vi "new DSF Configuration.vi"(8 "error in (no error)":errorcluster) -> (0 "error out":errorcluster, 3 "configuration cluster":T1)   [LabVIEW 2017, in "DSF Configuration API v1.0.0.lvlib"]
uses:
  DSF Configuration API v1.0.0.lvlib
  Controls/dsf configuration data/1.0.0/dsf configuration.ctl
  Controls/dsf configuration data/1.0.0/version.ctl
  Controls/dsf configuration data/1.0.0/dsf plugin.ctl
  Controls/dsf configuration data/1.0.0/dsf timing.ctl
  Controls/dsf configuration data/1.0.0/dsf group.ctl
  Controls/dsf configuration data/1.0.0/dsf transfer.ctl
  Controls/dsf configuration data/1.0.0/dsf channel.ctl
  Controls/dsf configuration data/1.0.0/dsf settings.ctl
  Controls/dsf configuration data/1.0.0/dsf configuration data v1.0.0.lvlib
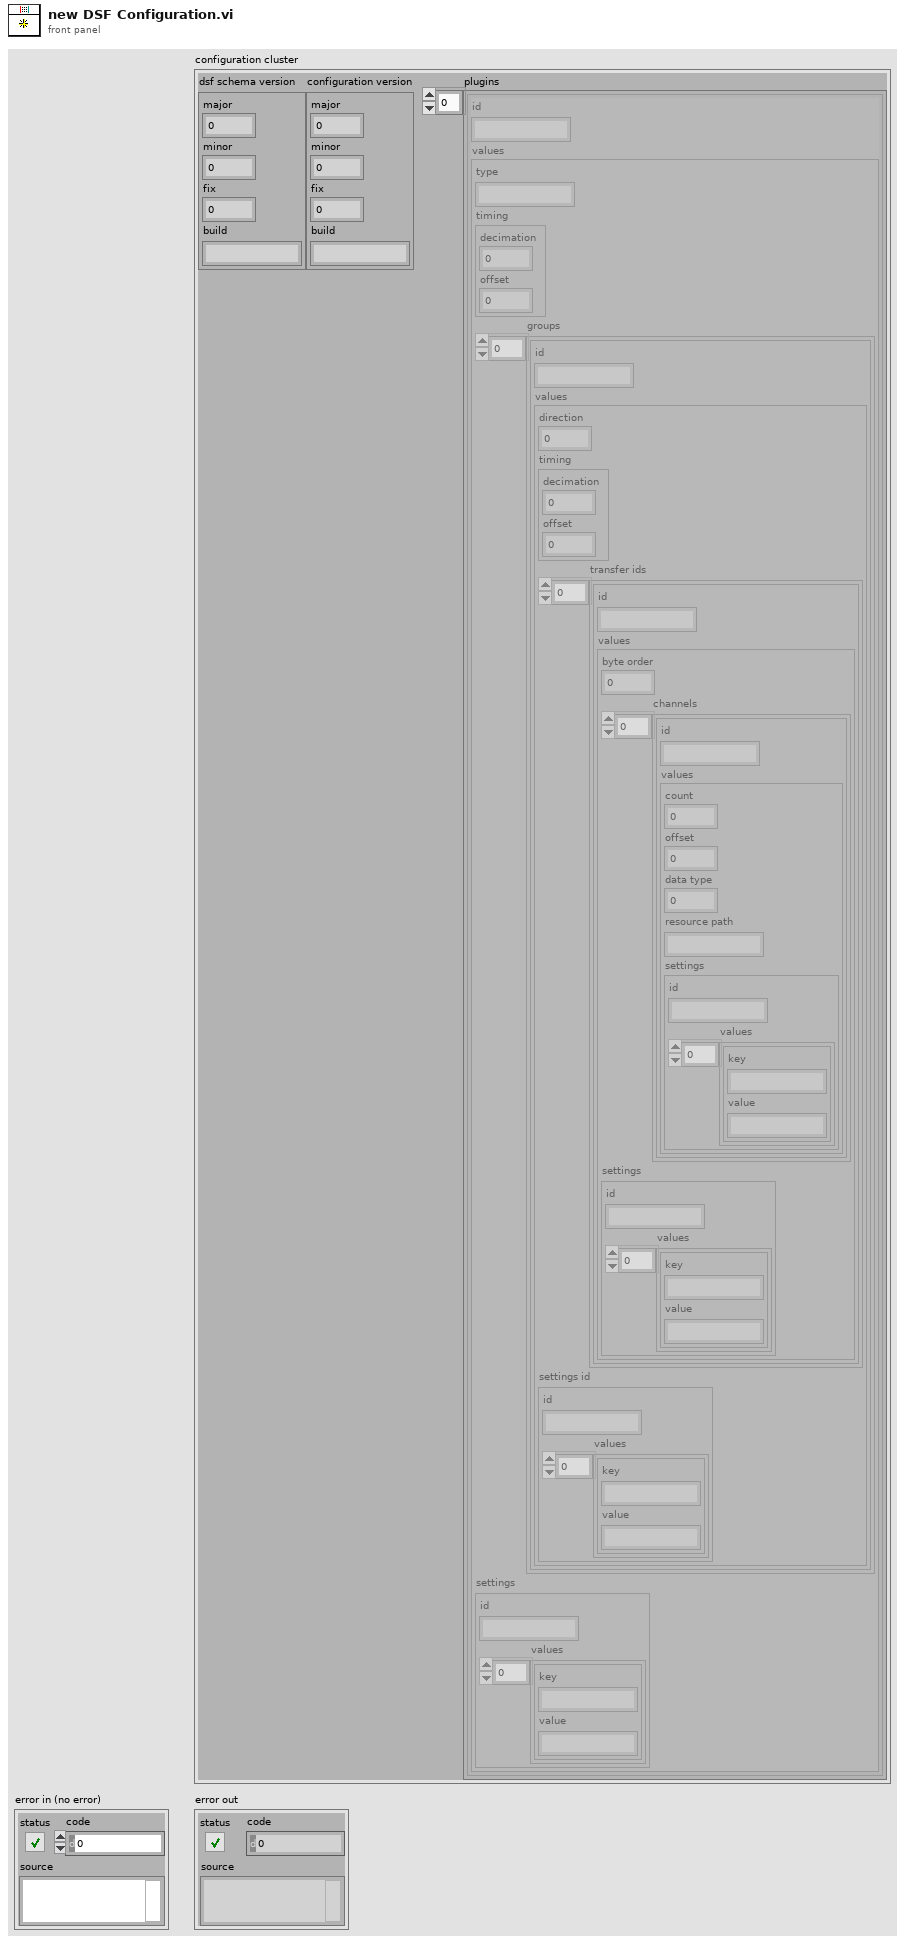
[diagram p1: front panel]
types:
  T1 = typedef "dsf configuration data v1.0.0.lvlib/dsf configuration.ctl" = cluster{"dsf schema version":T2, "configuration version":T2, "plugins":T3[]}
  T2 = typedef "dsf configuration data v1.0.0.lvlib/version.ctl" = cluster{"major":u32, "minor":u32, "fix":u32, "build":string}
  T3 = typedef "dsf configuration data v1.0.0.lvlib/dsf plugin.ctl" = cluster{"id":string, "values":cluster{"type":string, "timing":T4, "groups":T5[], "settings":T8}}
  T4 = typedef "dsf configuration data v1.0.0.lvlib/dsf timing.ctl" = cluster{"decimation":i32, "offset":i32}
  T5 = typedef "dsf configuration data v1.0.0.lvlib/dsf group.ctl" = cluster{"id":string, "values":cluster{"direction":i32, "timing":T4, "transfer ids":T6[], "settings id":T8}}
  T6 = typedef "dsf configuration data v1.0.0.lvlib/dsf transfer.ctl" = cluster{"id":string, "values":cluster{"byte order":i32, "channels":T7[], "settings":T8}}
  T7 = typedef "dsf configuration data v1.0.0.lvlib/dsf channel.ctl" = cluster{"id":string, "values":cluster{"count":i32, "offset":i32, "data type":i32, "resource path":string, "settings":T8}}
  T8 = typedef "dsf configuration data v1.0.0.lvlib/dsf settings.ctl" = cluster{"id":string, "values":cluster{"key":string, "value":string}[]}
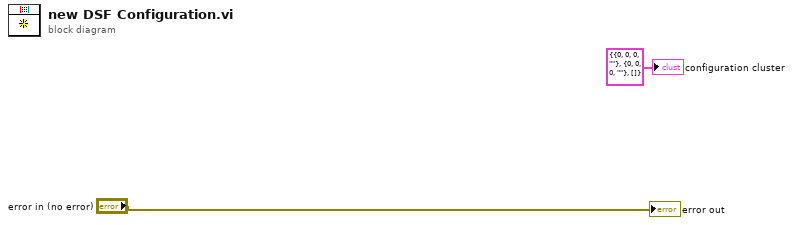
[diagram p0: block diagram]
diagram:
  "error out" <- "error in (no error)"
  "configuration cluster" <- T1 {"dsf schema version"={"major"=0, "minor"=0, "fix"=0, "build"=""}, "configuration version"={"major"=0, "minor"=0, "fix"=0, "build"=""}, "plugins"=[]} ("configuration cluster")
